vi "Kenimatics_VecBuilder_3x1Fill.vi"(9 "R2":dbl, 10 "R1":dbl, 11 "R0":dbl) -> (3 "output matrix":T1)   [LabVIEW 2023, in "Swerve_Odometry_SEN.lvlib"]
doc: "Build a 3 x 1 Matrix (vector) from an array of input values.\n\nInputs:\n -- R0 -- Input value 1\n -- R1 -- Input value 2\n -- R2 -- Input value 3\n\nOutputs:\n -- Output Matrix -- Resulting 3 x 1 matrix (vector)"
uses:
  Swerve_Odometry_SEN.lvlib
  <vilib>/Analysis/Matrix/Datatypes/RealMatrix.ctl
  <vilib>/Analysis/Matrix/NI_Matrix.lvlib
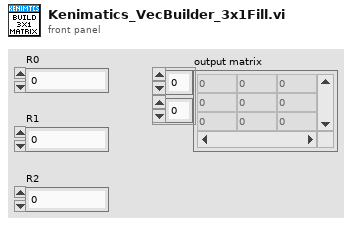
[diagram p1: front panel]
types:
  T1 = typedef "NI_Matrix.lvlib/RealMatrix.ctl" = dbl[][]
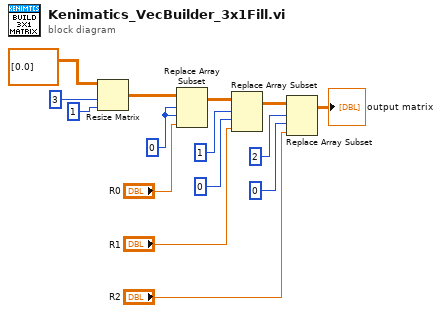
[diagram p0: block diagram]
diagram:
  w15 = 0 ("index (col)")
  n1 = Resize Matrix(1:1 ("Columns"), 2:3 ("Rows"), 4:T1 [[0.0]] ("matrix")) -> (0:w3:T1)
  n2 = Replace Array Subset(array=w3, new element="R0", index (row)=w15, index (col)=w15) -> (w13:T1)
  n3 = Replace Array Subset(array=w13, new element="R1", index (row)=1 ("index (col)"), index (col)=0 ("disabled index (col)")) -> (w6:T1)
  n4 = Replace Array Subset(array=w6, new element="R2", index (row)=2 ("index (col)"), index (col)=0 ("disabled index (col)")) -> (→"output matrix":T1)
